vi "LM Two H-Connected Gaussians and gradient.vi"(3 "output control":T1, 4 "data":variant, 5 "X":dbl[](array[numeric]), 6 "a":dbl[](array[numeric])) -> (0 "error out":errorcluster, 1 "f'(X,a)":dbl[][](array[numeric]), 2 "f(X,a)":dbl[](array[numeric]))   [LabVIEW 2019]
doc: "This template is the starting point for creating a model function to be passed to the Nonlinear Curve Fit.vi."
uses:
  <vilib>/gmath/NumericalOptimization/LM_output select.ctl
  D-Only Fixed Parameters.ctl
  <vilib>/gmath/NI_Gmath.lvlib
panel:
  # "Parameters:\n\nAmplitude 1: A1\nCenter 1: t1\nSDV 1: s1\nAmplitude 2: A2\nCenter 2: t2\nSDV 2: s2\n\nBridge Amplitude: A3"
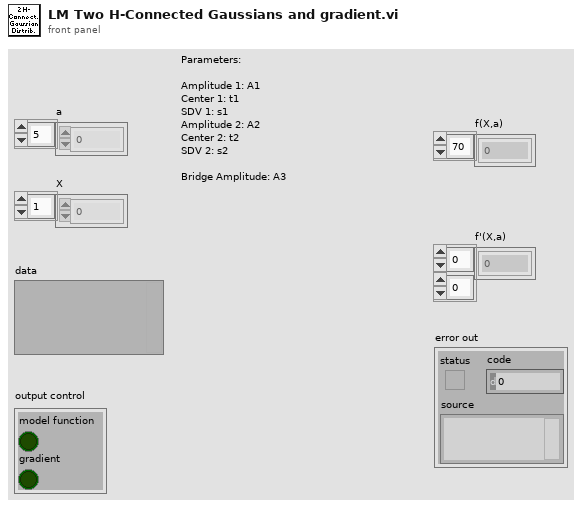
[diagram p1: front panel]
types:
  T1 = typedef "NI_Gmath.lvlib/LM_output select.ctl" = cluster{"model function":bool, "gradient":bool}
  T2 = typedef "D-Only Fixed Parameters.ctl" = cluster{"Fix D-only Peak Location":bool, "Peak Location":dbl, "Fix D-only Peak FWHM":bool, "Peak FWHM":dbl}
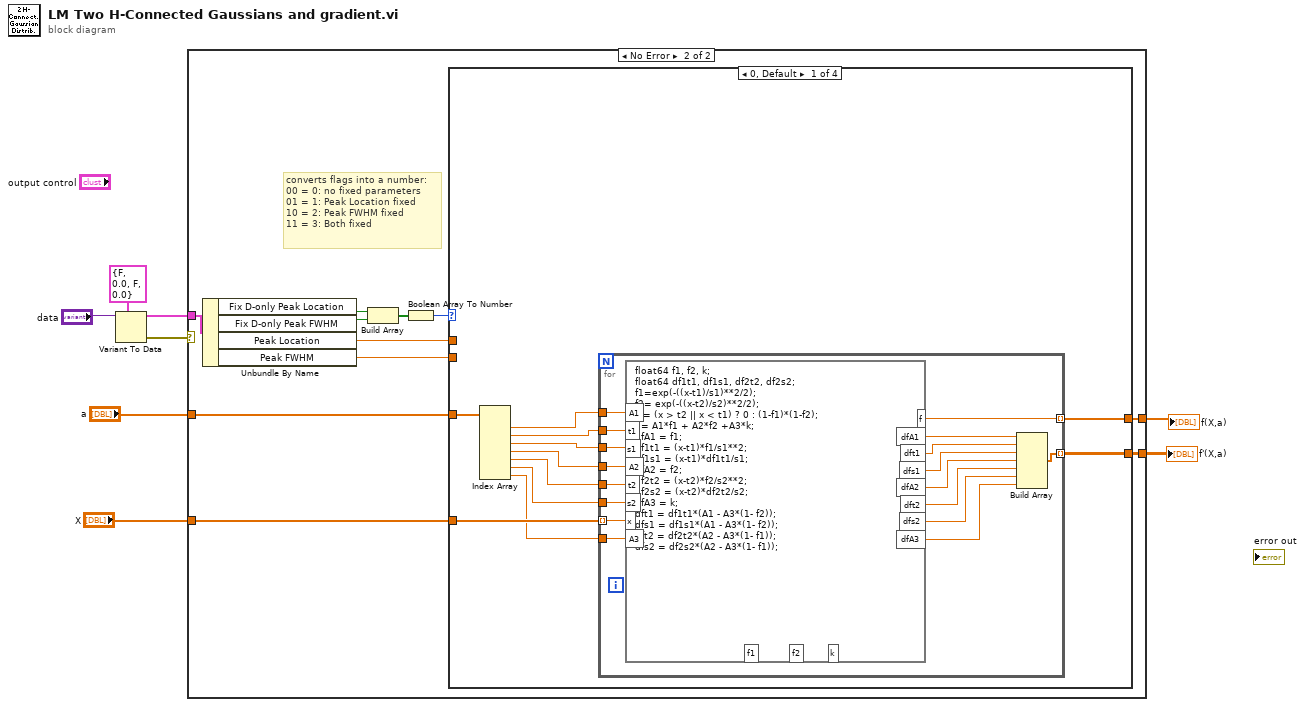
[diagram p0: block diagram]
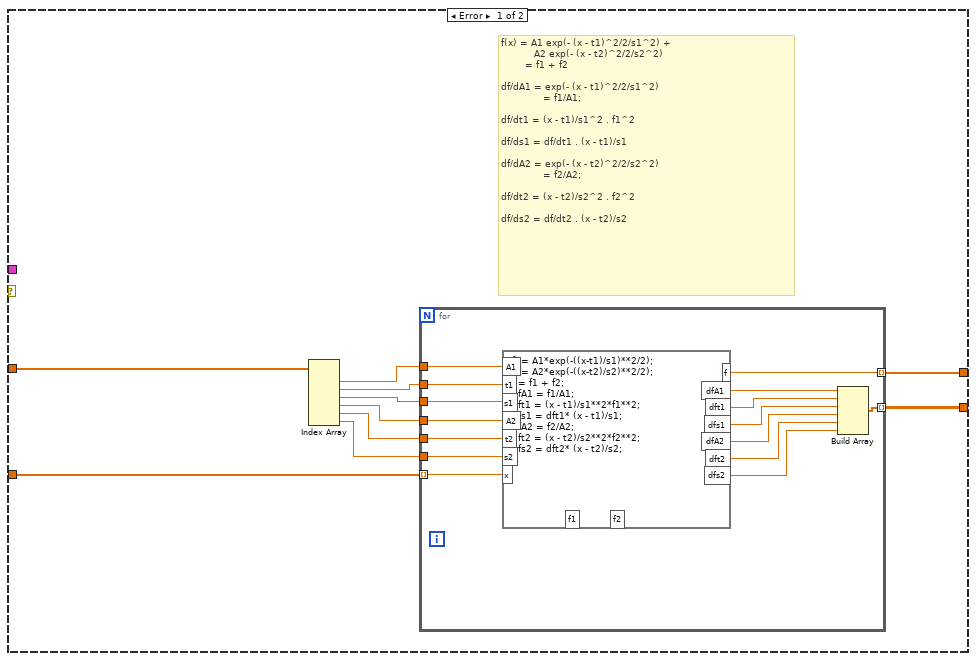
[diagram p2: hidden frame]
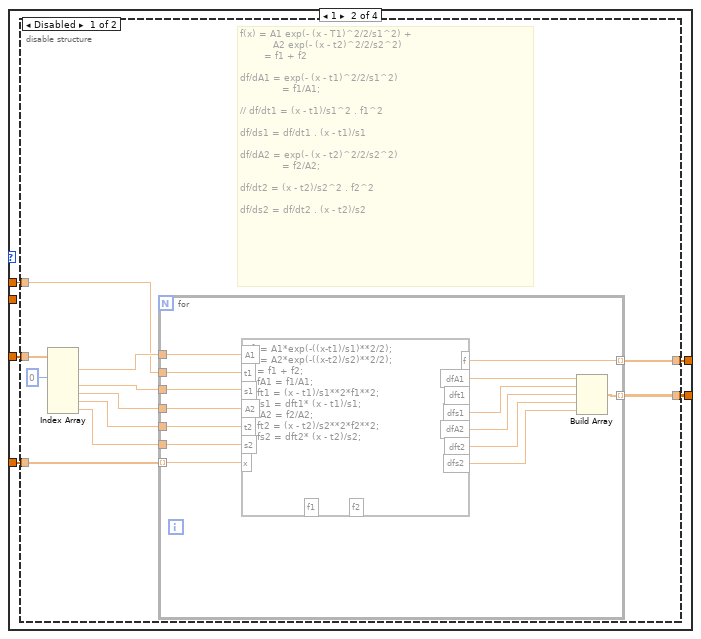
[diagram p3: hidden frame]
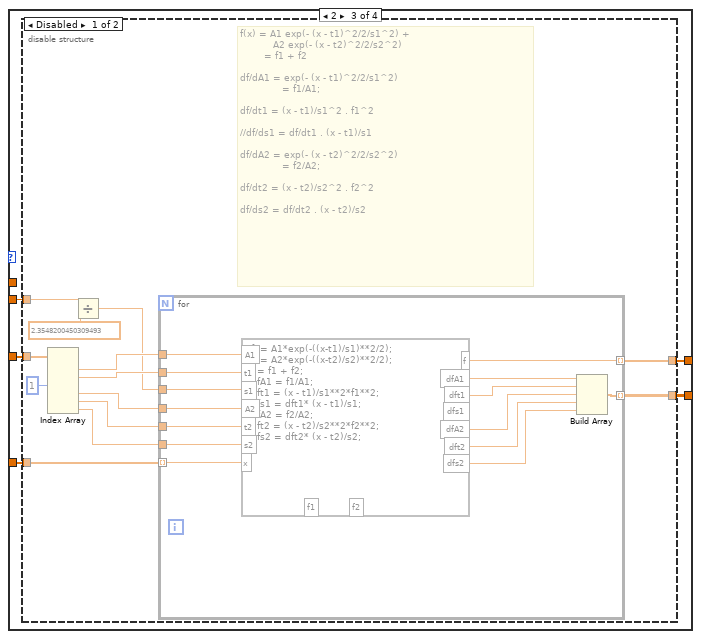
[diagram p5: hidden frame]
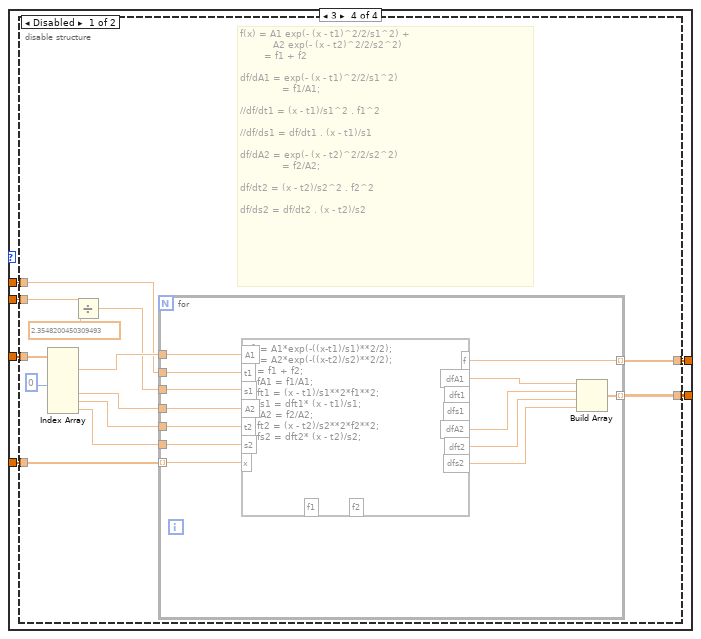
[diagram p7: hidden frame]
diagram:
  n1 = Variant To Data(type=T2 {"Fix D-only Peak Location"=FALSE, "Peak Location"=0.0, "Fix D-only Peak FWHM"=FALSE, "Peak FWHM"=0.0} ("Fixed Parameters"), Variant="data") -> (data=w1:T2, error out=w2:errorcluster)  [unwired: 1 in]
  n2 = case shown="No Error" w2 {
    tunnel: "a" -> [w18 w44]
    tunnel: "X" -> [w17 w43]
    tunnel: [w16 w42] -> w6
    tunnel: [w15 w41] -> w5
    tunnel: w1 -> [_ w40]
    frame Error {
      # "f(x) = A1 exp(- (x - t1)^2/2/s1^2) +\n           A2 exp(- (x - t2)^2/2/s2^2)\n        = f1 + f2\n\ndf/dA1 = exp(- (x - t1)^2/2/s1^2)\n              = f1/A1;\n\ndf/dt1 = (x - t1)/s1^2 . f1^2\n\ndf/ds1 = df/dt1 . (x - t1)/s1                     \n\ndf/dA2 = exp(- (x - t2)^2/2/s2^2)\n              = f2/A2;\n\ndf/dt2 = (x - t2)/s2^2 . f2^2\n\ndf/ds2 = df/dt2 . (x - t2)/s2"
      n3 = Index Array(array=w18) -> (element #1=w14:dbl, element #2=w13:dbl, element #3=w12:dbl, element #4=w11:dbl, element #5=w10:dbl, element #6=w9:dbl)  [unwired: 6 in]
      n4 = for {
        tunnel: w17 -> [w33] mode=indexing
        tunnel: [w31] -> w16 mode=indexing
        tunnel: [w30] -> w15 mode=indexing
        tunnel: w14 -> [w29]
        tunnel: w13 -> [w28]
        tunnel: w12 -> [w27]
        tunnel: w11 -> [w26]
        tunnel: w10 -> [w25]
        tunnel: w9 -> [w24]
        n5 = formula code="f1= A1*exp(-((x-t1)/s1)**2/2);\nf2= A2*exp(-((x-t2)/s2)**2/2);\nf = f1 + f2;\ndfA1 = f1/A1;\ndft1 = (x - t1)/s1**2*f1**2;\ndfs1 = dft1* (x - t1)/s1;\ndfA2 = f2/A2;\ndft2 = (x - t2)/s2**2*f2**2;\ndfs2 = dft2* (x - t2)/s2;"("A1"=w29, "t1"=w28, "s1"=w27, "x"=w33, "A2"=w26, "t2"=w25, "s2"=w24) -> ("f"=w31:dbl, "dfA1"=w32:dbl, "dft1"=w23:dbl, "dfs1"=w22:dbl, "dfA2"=w21:dbl, "dft2"=w20:dbl, "dfs2"=w19:dbl)  [unwired: 2 out]
        n6 = Build Array(w32, w23, w22, w21, w20, w19) -> (w30:dbl[])
      }
    }
    frame No Error {
      # "converts flags into a number:\n00 = 0: no fixed parameters\n01 = 1: Peak Location fixed\n10 = 2: Peak FWHM fixed\n11 = 3: Both fixed"
      n7 = Unbundle By Name(w40) -> ("Fix D-only Peak Location"=w39:bool, "Fix D-only Peak FWHM"=w38:bool, "Peak Location"=w35:dbl, "Peak FWHM"=w34:dbl)
      n8 = Build Array(w39, w38) -> (w37:bool[])
      n9 = Boolean Array To Number(Boolean array=w37) -> (number=w36:u32)
      n10 = case shown="0, Default" w36 {
        tunnel: w44 -> [w55 w77 w107 w140]
        tunnel: w43 -> [w54 w76 w106 w139]
        tunnel: [w53 w75 w105 w138] -> w42
        tunnel: [w52 w74 w104 w137] -> w41
        tunnel: w35 -> [_ w73 _ w135]
        tunnel: w34 -> [_ _ w103 w136]
        frame 0, Default {
          n11 = Index Array(array=w55) -> (element #1=w51:dbl, element #2=w50:dbl, element #3=w49:dbl, element #4=w48:dbl, element #5=w47:dbl, element #6=w46:dbl, element #7=w45:dbl)  [unwired: 7 in]
          n12 = for {
            tunnel: w54 -> [w72] mode=indexing
            tunnel: [w70] -> w53 mode=indexing
            tunnel: [w69] -> w52 mode=indexing
            tunnel: w51 -> [w68]
            tunnel: w50 -> [w67]
            tunnel: w49 -> [w66]
            tunnel: w48 -> [w65]
            tunnel: w47 -> [w64]
            tunnel: w46 -> [w63]
            tunnel: w45 -> [w57]
            n13 = formula code="float64 f1, f2, k;\nfloat64 df1t1, df1s1, df2t2, df2s2;\nf1=exp(-((x-t1)/s1)**2/2);\nf2= exp(-((x-t2)/s2)**2/2);\nk = (x > t2 || x < t1) ? 0 : (1-f1)*(1-f2);\nf = A1*f1 + A2*f2 +A3*k;\ndfA1 = f1;\ndf1t1 = (x-t1)*f1/s1**2;\ndf1s1 = (x-t1)*df1t1/s1;\ndfA2 = f2;\ndf2t2 = (x-t2)*f2/s2**2;\ndf2s2 = (x-t2)*df2t2/s2;\ndfA3 = k;\ndft1 = df1t1*(A1 - A3*(1- f2));\ndfs1 = df1s1*(A1 - A3*(1- f2));\ndft2 = df2t2*(A2 - A3*(1- f1));\ndfs2 = df2s2*(A2 - A3*(1- f1));"("A1"=w68, "t1"=w67, "s1"=w66, "x"=w72, "A2"=w65, "t2"=w64, "s2"=w63, "A3"=w57) -> ("f"=w70:dbl, "dfA1"=w71:dbl, "dft1"=w62:dbl, "dfs1"=w61:dbl, "dfA2"=w60:dbl, "dft2"=w59:dbl, "dfs2"=w58:dbl, "dfA3"=w56:dbl)  [unwired: 3 out]
            n14 = Build Array(w71, w62, w61, w60, w59, w58, w56) -> (w69:dbl[])
          }
        }
        frame 1 {
          n15 = disable-structure shown="Disabled" {
            disable-tunnel: w77 -> [w88 _]
            disable-tunnel: w76 -> [w87 _]
            disable-tunnel: [w86 _] -> w75
            disable-tunnel: [w85 _] -> w74
            disable-tunnel: w73 -> [w79 _]
            frame Disabled {
              # "f(x) = A1 exp(- (x - T1)^2/2/s1^2) +\n           A2 exp(- (x - t2)^2/2/s2^2)\n        = f1 + f2\n\ndf/dA1 = exp(- (x - t1)^2/2/s1^2)\n              = f1/A1;\n\n// df/dt1 = (x - t1)/s1^2 . f1^2\n\ndf/ds1 = df/dt1 . (x - t1)/s1                     \n\ndf/dA2 = exp(- (x - t2)^2/2/s2^2)\n              = f2/A2;\n\ndf/dt2 = (x - t2)/s2^2 . f2^2\n\ndf/ds2 = df/dt2 . (x - t2)/s2"
              n16 = Index Array(array=w88, index #2=0 ("index")) -> (element #1=w84:dbl, element #3=w83:dbl, element #4=w82:dbl, element #5=w81:dbl, element #6=w80:dbl)  [unwired: 5 in, 1 out]
              n17 = for {
                tunnel: w87 -> [w102] mode=indexing
                tunnel: [w100] -> w86 mode=indexing
                tunnel: [w99] -> w85 mode=indexing
                tunnel: w84 -> [w98]
                tunnel: w79 -> [w97]
                tunnel: w83 -> [w96]
                tunnel: w82 -> [w95]
                tunnel: w81 -> [w94]
                tunnel: w80 -> [w93]
                n18 = formula code="f1= A1*exp(-((x-t1)/s1)**2/2);\nf2= A2*exp(-((x-t2)/s2)**2/2);\nf = f1 + f2;\ndfA1 = f1/A1;\ndft1 = (x - t1)/s1**2*f1**2;\ndfs1 = dft1* (x - t1)/s1;\ndfA2 = f2/A2;\ndft2 = (x - t2)/s2**2*f2**2;\ndfs2 = dft2* (x - t2)/s2;"("A1"=w98, "t1"=w97, "s1"=w96, "x"=w102, "A2"=w95, "t2"=w94, "s2"=w93) -> ("f"=w100:dbl, "dfA1"=w101:dbl, "dfs1"=w92:dbl, "dfA2"=w91:dbl, "dft2"=w90:dbl, "dfs2"=w89:dbl)  [unwired: 3 out]
                n19 = Build Array(w101, w92, w91, w90, w89) -> (w99:dbl[])
              }
            }
            frame Enabled {
            }
          }
        }
        frame 2 {
          n20 = disable-structure shown="Disabled" {
            disable-tunnel: w107 -> [w120 _]
            disable-tunnel: w106 -> [w119 _]
            disable-tunnel: [w118 _] -> w105
            disable-tunnel: [w117 _] -> w104
            disable-tunnel: w103 -> [w111 _]
            frame Disabled {
              # "f(x) = A1 exp(- (x - t1)^2/2/s1^2) +\n           A2 exp(- (x - t2)^2/2/s2^2)\n        = f1 + f2\n\ndf/dA1 = exp(- (x - t1)^2/2/s1^2)\n              = f1/A1;\n\ndf/dt1 = (x - t1)/s1^2 . f1^2\n\n//df/ds1 = df/dt1 . (x - t1)/s1                     \n\ndf/dA2 = exp(- (x - t2)^2/2/s2^2)\n              = f2/A2;\n\ndf/dt2 = (x - t2)/s2^2 . f2^2\n\ndf/ds2 = df/dt2 . (x - t2)/s2"
              n21 = Index Array(array=w120, index #3=1 ("index")) -> (element #1=w116:dbl, element #2=w115:dbl, element #4=w114:dbl, element #5=w113:dbl, element #6=w112:dbl)  [unwired: 5 in, 1 out]
              n22 = Divide(x=w111, y=2.3548200450309493) -> (x/y=w109:dbl)
              n23 = for {
                tunnel: w119 -> [w134] mode=indexing
                tunnel: [w132] -> w118 mode=indexing
                tunnel: [w131] -> w117 mode=indexing
                tunnel: w116 -> [w130]
                tunnel: w115 -> [w129]
                tunnel: w109 -> [w128]
                tunnel: w114 -> [w127]
                tunnel: w113 -> [w126]
                tunnel: w112 -> [w125]
                n24 = formula code="f1= A1*exp(-((x-t1)/s1)**2/2);\nf2= A2*exp(-((x-t2)/s2)**2/2);\nf = f1 + f2;\ndfA1 = f1/A1;\ndft1 = (x - t1)/s1**2*f1**2;\ndfs1 = dft1* (x - t1)/s1;\ndfA2 = f2/A2;\ndft2 = (x - t2)/s2**2*f2**2;\ndfs2 = dft2* (x - t2)/s2;"("A1"=w130, "t1"=w129, "s1"=w128, "x"=w134, "A2"=w127, "t2"=w126, "s2"=w125) -> ("f"=w132:dbl, "dfA1"=w133:dbl, "dft1"=w124:dbl, "dfA2"=w123:dbl, "dft2"=w122:dbl, "dfs2"=w121:dbl)  [unwired: 3 out]
                n25 = Build Array(w133, w124, w123, w122, w121) -> (w131:dbl[])
              }
            }
            frame Enabled {
            }
          }
        }
        frame 3 {
          n26 = disable-structure shown="Disabled" {
            disable-tunnel: w140 -> [w153 _]
            disable-tunnel: w139 -> [w152 _]
            disable-tunnel: [w151 _] -> w138
            disable-tunnel: [w150 _] -> w137
            disable-tunnel: w136 -> [w145 _]
            disable-tunnel: w135 -> [w142 _]
            frame Disabled {
              # "f(x) = A1 exp(- (x - t1)^2/2/s1^2) +\n           A2 exp(- (x - t2)^2/2/s2^2)\n        = f1 + f2\n\ndf/dA1 = exp(- (x - t1)^2/2/s1^2)\n              = f1/A1;\n\n//df/dt1 = (x - t1)/s1^2 . f1^2\n\n//df/ds1 = df/dt1 . (x - t1)/s1                     \n\ndf/dA2 = exp(- (x - t2)^2/2/s2^2)\n              = f2/A2;\n\ndf/dt2 = (x - t2)/s2^2 . f2^2\n\ndf/ds2 = df/dt2 . (x - t2)/s2"
              n27 = Index Array(array=w153, index #3=0 ("index")) -> (element #1=w149:dbl, element #4=w148:dbl, element #5=w147:dbl, element #6=w146:dbl)  [unwired: 5 in, 2 out]
              n28 = Divide(x=w145, y=2.3548200450309493) -> (x/y=w143:dbl)
              n29 = for {
                tunnel: w152 -> [w166] mode=indexing
                tunnel: [w164] -> w151 mode=indexing
                tunnel: [w163] -> w150 mode=indexing
                tunnel: w149 -> [w162]
                tunnel: w142 -> [w161]
                tunnel: w143 -> [w160]
                tunnel: w148 -> [w159]
                tunnel: w147 -> [w158]
                tunnel: w146 -> [w157]
                n30 = formula code="f1= A1*exp(-((x-t1)/s1)**2/2);\nf2= A2*exp(-((x-t2)/s2)**2/2);\nf = f1 + f2;\ndfA1 = f1/A1;\ndft1 = (x - t1)/s1**2*f1**2;\ndfs1 = dft1* (x - t1)/s1;\ndfA2 = f2/A2;\ndft2 = (x - t2)/s2**2*f2**2;\ndfs2 = dft2* (x - t2)/s2;"("A1"=w162, "t1"=w161, "s1"=w160, "x"=w166, "A2"=w159, "t2"=w158, "s2"=w157) -> ("f"=w164:dbl, "dfA1"=w165:dbl, "dfA2"=w156:dbl, "dft2"=w155:dbl, "dfs2"=w154:dbl)  [unwired: 4 out]
                n31 = Build Array(w165, w156, w155, w154) -> (w163:dbl[])
              }
            }
            frame Enabled {
            }
          }
        }
      }
    }
  }
  "f(X,a)" <- w6
  "f'(X,a)" <- w5
